vi "Save DAC Configuration.vi"(8 "error in":errorcluster, 10 "Config File refnum in":T1, 11 "DAC HeatFlow Temp in":refnum<class "DAC RTD Temp.lvclass">) -> (0 "error out":errorcluster, 2 "Config File refnum out":T1, 3 "DAC HeatFlow Temp out":refnum<class "DAC RTD Temp.lvclass">)   [LabVIEW 2019, in "DAC.lvlib" / "DAC RTD Temp.lvclass"]
uses:
  DAC RTD Temp.lvclass
  C:/Users/wg/Documents/LV_Projects/test-stand/App/DAC/DAC.lvclass
  <vilib>/Utility/config.llb/Config Data RefNum.ctl
  DAC.lvclass/DAC.ctl
  DAC RTD Temp.lvclass/DAC RTD Temp.ctl
  <vilib>/Utility/config.llb/Write Key (String).vi
  DAC.lvclass
  <vilib>/Utility/config.llb/NI_LVConfig.lvlib
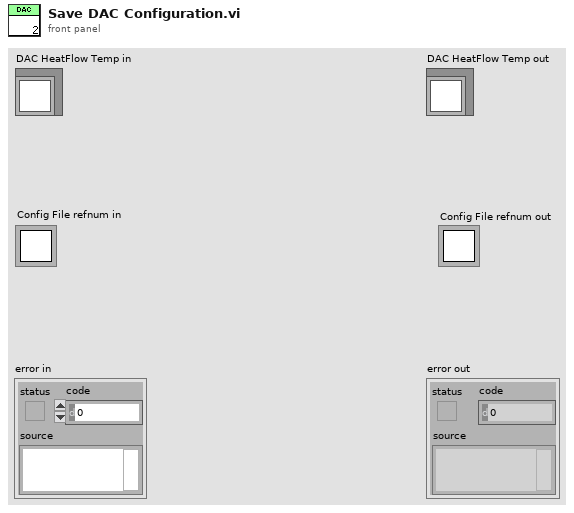
[diagram p1: front panel]
types:
  T1 = typedef "NI_LVConfig.lvlib/Config Data RefNum.ctl" = refnum<k1>
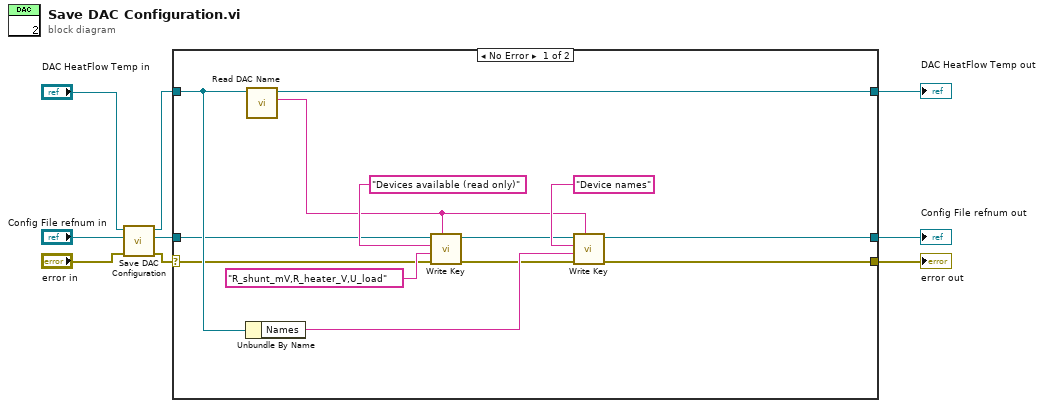
[diagram p0: block diagram]
diagram:
  n1 = call-parent "Save DAC Configuration.vi"("error in"="error in", "Config File refnum in"="Config File refnum in", "DAC in"="DAC HeatFlow Temp in") -> ("error out"=w4:errorcluster, "Config File refnum out"=w5:T1, "DAC out"=w6:refnum<class "DAC RTD Temp.lvclass">)  [unwired: 6 in]
  n2 = case shown="No Error" w4 {
    selector: w4 -> [w15 w25]
    tunnel: [w11 w25] -> w1
    tunnel: [w20 w24] -> w3
    tunnel: w6 -> [w21 w24]
    tunnel: w5 -> [w14 w23]
    tunnel: [w12 w23] -> w2
    frame No Error {
      n3 = Unbundle By Name(w21) -> ("Names"=w19:string)
      n4 = call "Read DAC Name.vi"("DAC in"=w21) -> ("DAC Name"=w10:string, "DAC out"=w20:refnum<class "DAC RTD Temp.lvclass">)  [unwired: 8 in, 1 out]
      n5 = call-poly <vilib>:"Write Key.vi"("section"=w10, "error in (no error)"=w15, "value"="R_shunt_mV,R_heater_V,U_load", "key"="Devices available (read only)", "refnum"=w14) -> ("error out"=w16:errorcluster, "refnum out"=w13:T1)  [unwired: 4 in, 1 out]
      n6 = call-poly <vilib>:"Write Key.vi"("section"=w10, "error in (no error)"=w16, "value"=w19, "key"="Device names", "refnum"=w13) -> ("error out"=w11:errorcluster, "refnum out"=w12:T1)  [unwired: 4 in, 1 out]
    }
    frame Error {
    }
  }
  "error out" <- w1
  "DAC HeatFlow Temp out" <- w3
  "Config File refnum out" <- w2
